vi "Timestamp or now.vi"(1 "timestamp (now)":timestamp) -> (0 "timestamp":timestamp)   [LabVIEW 2019]
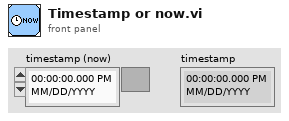
[diagram p1: front panel]
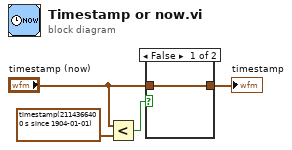
[diagram p0: block diagram]
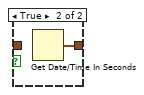
[diagram p2: hidden frame]
diagram:
  n1 = Less?(x="timestamp (now)", y=timestamp(2114366400 s since 1904-01-01) ("timestamp (now)")) -> (x < y?=w2:bool)
  n2 = case shown="False" w2 {
    tunnel: [w5 w6] -> w3
    tunnel: "timestamp (now)" -> [w5 _]
    frame False {
    }
    frame True {
      n3 = Get Date/Time In Seconds() -> (seconds since 1Jan1904=w6:timestamp)
    }
  }
  "timestamp" <- w3
